vi "AP2_photoelectron_image_aquisition.vi"() -> ()   [LabVIEW 2023]
panel:
  in  "Tab Control 2":enum32{"Image Slice"}(tab)
  out "Image Slice":dbl[](graph)
  in  "Calc R pixel":bool
  in  "Center Y":dbl=555.0
  in  "Center X":dbl=548.0
  in  "Tab Control":enum32{"PES Acquisition Controls and Montoring"}(tab)
  out "B Counts/5F":dbl
  out "Avg Counts/F":dbl
  out "A Counts":u32
  out "B Counts":u32
  out "Total Counts":u32
  out "A Counts/5F":dbl
  in  "Stop Control":bool
  in  "Save Image Button":bool
  in  "Discard Image Button":bool
  in  "Threshold range":cluster{"Lower value":sgl, "Upper value":sgl}={"Lower value"=6.0, "Upper value"=1024.0}
  in  "Region of interest":i32[](array[numeric])
  in  "Number of buffers":u32
  in  "Frame timeout (ms)":u32=1000
  in  "Update img":bool
  out "FPS":dbl
  out "Processing time / ms":u32
  out "Accumulated Image":i16[][](graph)
  # "Monitoring"
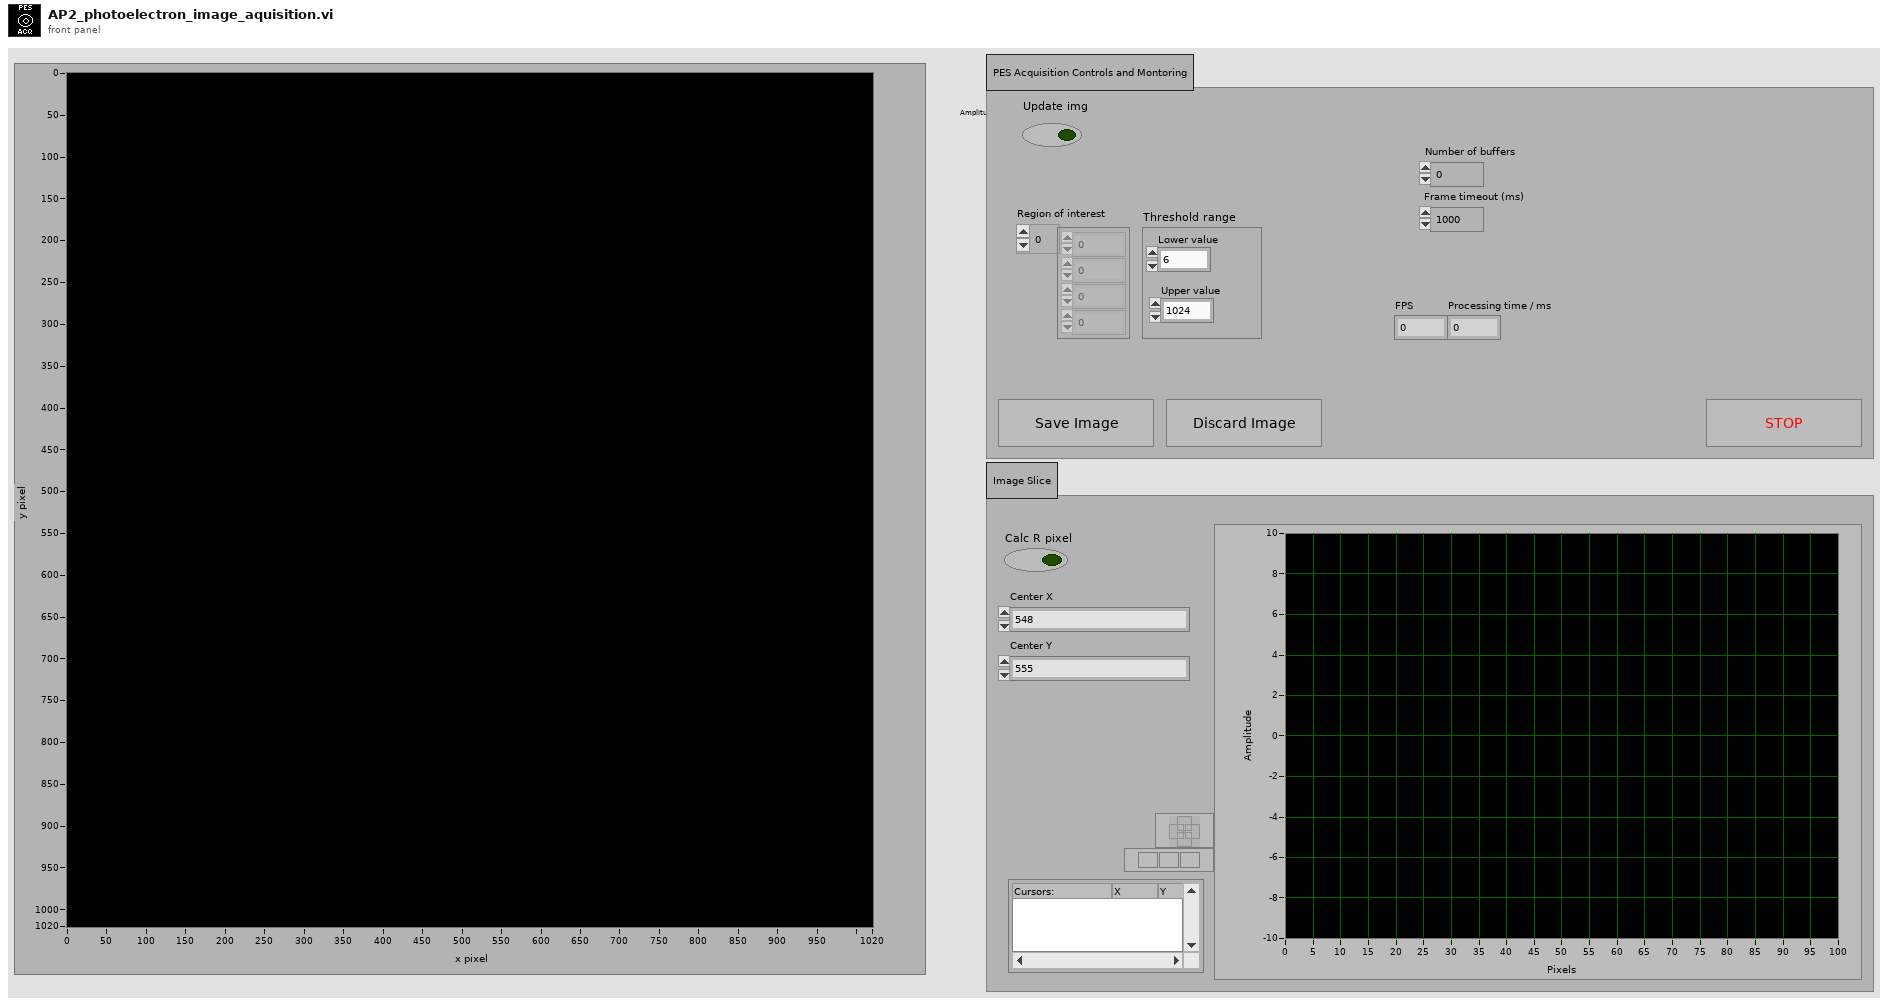
[diagram p1: front panel]
types:
  T1 = cluster{"Region of interest":i32[], "Number of buffers":u32, "Frame timeout (ms)":u32}
  T2 = cluster{"queue out":refnum<queue>, "error out":errorcluster}
  T3 = cluster{"i01 data":sgl[][], "i02 data":sgl[][], "Count Buffer Size Out":i32, "Empty Image":i16[][], "Accumulated Image":i16[][], "Corrected Image 1":i16[][], "Corrected Image 2":i16[][], "Total counts":i32, "t_1":i32, "t_2":i32, "t_3":i32, "t_4":i32, "t_5":i32, "t_6":i32, "t_7":i32, "t_8":i32, "t_9":i32, "t_10":i32, "c_1":i32, "c_2":i32, "Region of interest":i32[]}
  T4 = cluster{"Total Counts":u32, "Avg Counts/F":dbl, "B Counts":u32, "A Counts":u32, "A Counts/5F":dbl, "B Counts/5F":dbl}
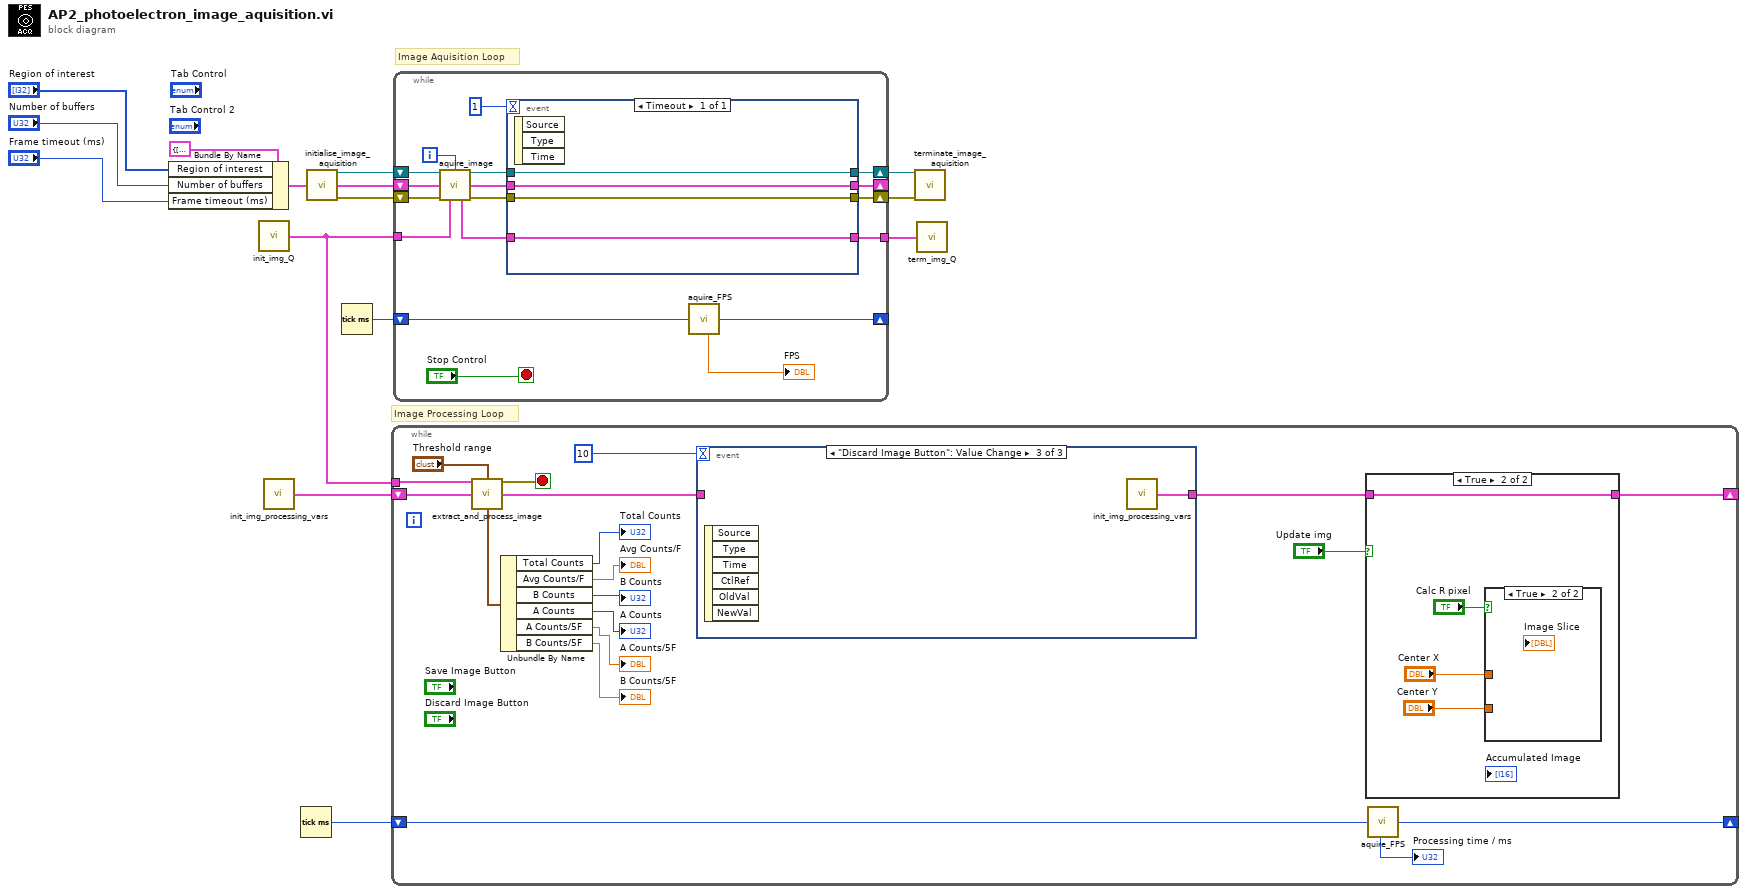
[diagram p0: block diagram]
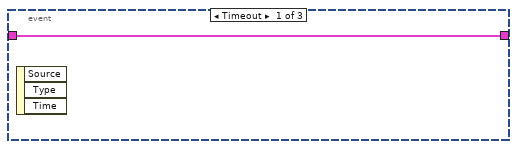
[diagram p2: hidden frame]
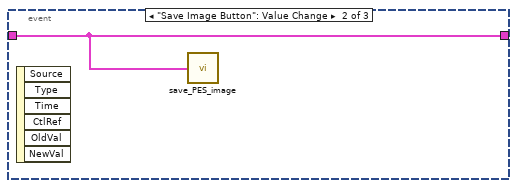
[diagram p3: hidden frame]
diagram:
  # "Image Processing Loop"
  # "Image Aquisition Loop"
  n1 = Bundle By Name(cluster=T1 {"Region of interest"=[], "Number of buffers"=0, "Frame timeout (ms)"=1000}, "Region of interest"="Region of interest", "Number of buffers"="Number of buffers", "Frame timeout (ms)"="Frame timeout (ms)") -> (w9:T1)
  n2 = call "init_img_Q.vi"() -> ("Image Q Out"=w6:T2)  [unwired: 15 in]
  n3 = call "init_img_processing_vars.vi"() -> ("Image Processing Data"=w2:T3)  [unwired: 15 in]
  n4 = Tick Count (ms)() -> (millisecond timer value=w3:u32)
  n5 = call "initialise_image_aquisition.vi"("Imaging Variables In"=w9) -> ("IMAQ Session Out"=w15:refnum<k11>, "Imaging Variables Out"=w8:T1, "error out"=w14:errorcluster)  [unwired: 11 in, 1 out]
  n6 = Tick Count (ms)() -> (millisecond timer value=w1:u32)
  n7 = while {
    tunnel: w6 -> [w31]
    shift-right: [w32] -> _
    shift-left: w3 -> [w33]
    shift-right: [w28] -> _
    shift-left: w2 -> [w29]
    stop <- w30 stop-if-true
    n8 = call "extract_and_process_image.vi"("Image Q In"=w31, "Threshold range"="Threshold range", "Processed Image Data In"=w29) -> ("error out"=w30:errorcluster, "Processed Image Data Out"=w26:T3, "Count data"=w23:T4)  [unwired: 10 in]
    n9 = Unbundle By Name(w23) -> ("Total Counts"=→"Total Counts":u32, "Avg Counts/F"=→"Avg Counts/F":dbl, "B Counts"=→"B Counts":u32, "A Counts"=→"A Counts":u32, "A Counts/5F"=→"A Counts/5F":dbl, "B Counts/5F"=→"B Counts/5F":dbl)
    n10 = event shown="[2] \"Discard Image Button\": Value Change" {
      selector: _ -> [_ _ _]
      dyn-events: _ -> [_ _ _]
      timeout: 10 -> [_ _ _]
      tunnel: w26 -> [w35 w36 _]
      tunnel: [w35 w36 w37] -> w24
      event Timeout {
        n11 = event-data() -> ()  [unwired: 1 in, 3 out]
      }
      event "Save Image Button": Value Change {
        n12 = event-data() -> ()  [unwired: 1 in, 6 out]
        n13 = call "save_PES_image.vi"("Processed Image Data In"=w36) -> ()  [unwired: 15 in]
      }
      event "Discard Image Button": Value Change {
        n14 = event-data() -> ()  [unwired: 1 in, 6 out]
        n15 = call "init_img_processing_vars.vi"() -> ("Image Processing Data"=w37:T3)  [unwired: 15 in]
      }
    }
    n16 = case shown="True" "Update img" {
      tunnel: w24 -> [w38 w39]
      tunnel: [w38 w39] -> w28
      frame False {
      }
      frame True {
        n17 = case shown="True" "Calc R pixel" {
          tunnel: "Center X" -> [_ _]
          tunnel: "Center Y" -> [_ _]
          frame False {
          }
          frame True {
          }
        }
      }
    }
    n18 = call "aquire_FPS.vi"("Time Value In /ms"=w33) -> ("Time Value Out /ms"=w32:u32, "Execution time / ms"=→"Processing time / ms":u32)  [unwired: 12 in, 1 out]
  }
  n19 = while {
    shift-right: [w59] -> w5
    shift-left: w15 -> [w56]
    shift-right: [w57] -> w4
    shift-left: w14 -> [w55]
    tunnel: w6 -> [w48]
    tunnel: [w47] -> w7
    shift-right: [w58] -> _
    shift-left: w8 -> [w51]
    shift-right: [w43] -> _
    shift-left: w1 -> [w45]
    i -> [w54]
    stop <- "Stop Control" stop-if-true
    n20 = call "aquire_image.vi"("IMAQ Session In"=w56, "Buffer to extract"=w54, "Imaging Variables In"=w51, "error in (no error)"=w55, "Img Q Data In"=w48) -> ("IMAQ Session Out"=w53:refnum<k11>, "Imaging Variables Out"=w50:T1, "Img Q Data Out"=w49:T2, "error out"=w52:errorcluster)  [unwired: 7 in]
    n21 = event shown="[0] Timeout" {
      selector: _ -> [_]
      dyn-events: _ -> [_]
      timeout: 1 -> [_]
      tunnel: w53 -> [w64]
      tunnel: w52 -> [w63]
      tunnel: [w64] -> w59
      tunnel: [w63] -> w57
      tunnel: w50 -> [w62]
      tunnel: [w62] -> w58
      tunnel: w49 -> [w61]
      tunnel: [w61] -> w47
      event Timeout {
        n22 = event-data() -> ()  [unwired: 1 in, 3 out]
      }
    }
    n23 = call "aquire_FPS.vi"("Time Value In /ms"=w45) -> ("Time Value Out /ms"=w43:u32, "FPS"=→"FPS":dbl)  [unwired: 12 in, 1 out]
  }
  n24 = call "terminate_image_aquisition.vi"("IMAQ Session In"=w5, "error in (no error)"=w4) -> ()  [unwired: 13 in, 1 out]
  n25 = call "term_img_Q.vi"("Image Q Out"=w7) -> ()  [unwired: 14 in, 1 out]
